vi "Begin.vi"(8 "error in":errorcluster) -> (0 "error out":errorcluster)   [LabVIEW 2018]
doc: "Called before other user functions, this VI is expected to open initial I/O refnums, load in file data, and do all program initialization. Notice that the <B>error out</B> terminal is simply used for data flow. Wiring it to other structures or subVIs ensures that this VI runs first."
uses:
  <vilib>/Rock Robotics/WPI/DriverStation/WPI_DriverStationRobotMode2.ctl
  <vilib>/Rock Robotics/WPI/Joystick/WPI_JoystickDeviceEnum.ctl
  <vilib>/Rock Robotics/WPI/Solenoid/WPI_SolenoidChannel.ctl
  <vilib>/Rock Robotics/WPI/ThirdParty/Phoenix-LabVIEW/Motor Controller/Controls/CTRE_Phoenix_MotorControl_ControlMode.ctl
  <vilib>/Rock Robotics/WPI/SafetyOutput/WPI_SafetyOutputConfigMenu.ctl
  <vilib>/Rock Robotics/SystemInterfaces/DIO/FPGA_DIOChannel.ctl
  Robot Global Data.vi
  <vilib>/Rock Robotics/Network Tables/NT Write String Array.vi
  <vilib>/Rock Robotics/WPI/Solenoid/WPI_SolenoidOpenSingle.vi
  <vilib>/Rock Robotics/WPI/RobotDrive/WPI_RobotDriveOpen2MotorWithExistingMotors.vi
  <vilib>/Rock Robotics/WPI/RobotDrive/WPI_RobotDriveOpen4MotorWithExistingMotors.vi
  <vilib>/Rock Robotics/WPI/Counter/WPI_CounterDigitalInputToDigitalSource.vi
  <vilib>/Rock Robotics/WPI/Utilities/WPI_GetSetVariantRefNum.vi
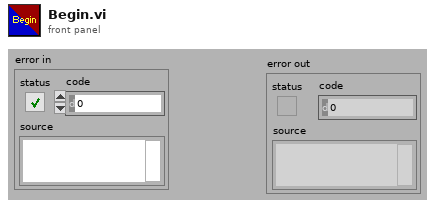
[diagram p1: front panel]
types:
  T1 = typedef "FPGA_DIOChannel.ctl" = enum8{"DIO 0", "DIO 1", "DIO 2", "DIO 3", "DIO 4", "DIO 5", "DIO 6", "DIO 7", "DIO 8", "DIO 9", "DIO MXP 0", "DIO MXP 1", "DIO MXP 2", "DIO MXP 3", "DIO MXP 4", "DIO MXP 5", "DIO MXP 6", "DIO MXP 7", "DIO MXP 8", "DIO MXP 9", "DIO MXP 10", "DIO MXP 11", "DIO MXP 12", "DIO MXP 13", "DIO MXP 14", "DIO MXP 15", "SPI Port CS1", "SPI Port CS2", "SPI Port CS3", "SPI Port MISO", "SPI Port MOSI", "Invalid"}
  T2 = typedef "CTRE_Phoenix_MotorControl_ControlMode.ctl" = u16
  T3 = typedef "WPI_SafetyOutputConfigMenu.ctl" = enum16{"Enable", "Disable"}
  T4 = typedef "WPI_JoystickDeviceEnum.ctl" = enum16{"USB 0", "USB 1", "USB 2", "USB 3", "USB 4", "USB 5"}
  T5 = typedef "WPI_SolenoidChannel.ctl" = enum8{"Solenoid 0", "Solenoid 1", "Solenoid 2", "Solenoid 3", "Solenoid 4", "Solenoid 5", "Solenoid 6", "Solenoid 7", "Invalid"}
  T6 = typedef "WPI_DriverStationRobotMode2.ctl" = enum16{"Autonomous Disabled", "Autonomous Enabled", "Teleop Disabled", "Teleop Enabled", "Disconnected", "Finish", "Test Disabled", "Test Enabled", "Emergency Stopped"}
  T7 = typedef "WPI_MotorControlDeviceRef.ctl" = cluster{"DeviceStatus":errorcluster, "Type":T8, "PWM":cluster{"PWM Channel":T9, "DeadBand":T10}, "CAN":cluster{"Device Number":u8, "SetOutput VI Ref":variant, "GetOutput VI Ref":variant, "Enable VI Ref":variant, "Disable VI Ref":variant, "Data":variant}, "Invert":bool, "DIO PWM":cluster{"PWM \"Enable\" Channel":T9, "DIOChannel":T1, "PWM Rate":dbl}}
  T8 = typedef "WPI_MotorControlType.ctl" = enum16{"PWM", "CAN", "DIO PWM"}
  T9 = typedef "FPGA_DIOPWMChannel.ctl" = enum8{"PWM 0", "PWM 1", "PWM 2", "PWM 3", "PWM 4", "PWM 5", "PWM 6", "PWM 7", "PWM 8", "PWM 9", "PWM MXP 0", "PWM MXP 1", "PWM MXP 2", "PWM MXP 3", "PWM MXP 4", "PWM MXP 5", "PWM MXP 6", "PWM MXP 7", "PWM MXP 8", "PWM MXP 9", "Invalid"}
  T10 = typedef "WPI_PWMDeadband.ctl" = cluster{"Name":string, "maxPositivePwm":i32, "minPositivePwm":i32, "centerPwm":i32, "maxNegativePwm":i32, "minNegativePwm":i32, "angularRange":u16}
  T11 = typedef "WPI_RobotDriveDevRef.ctl" = cluster{"DevStatus":errorcluster, "Motors[]":T7[], "Square Inputs":bool, "Max Output":dbl}
  T12 = typedef "WPI_CompressorDevRef.ctl" = cluster{"DevStatus":errorcluster, "Pneumatics Control Module":u8}
  T13 = typedef "WPI_JoystickDevRef.ctl" = cluster{"Device":T4}
  T14 = typedef "WPI_DigitalInputDevRef.ctl" = cluster{"DevStatus":errorcluster, "DIO Channel":T1}
  T15 = typedef "WPI_SolenoidDevRef.ctl" = cluster{"DevStatus":errorcluster, "Pneumatics Control Module":u8, "Forward Solenoid Channel":T5, "Reverse Solenoid Channel":T5}
  T16 = typedef "FPGA_CounterEncoderSourceConvertionLVSourceType.ctl" = cluster{"DevStatus":errorcluster, "AnalogTriggerMode?":bool, "DigitalMode":cluster{"DIO Channel":T17}, "AnalogTriggerMode":cluster{"AnalogTriggerIndex":T18, "OutputType":T19}}
  T17 = typedef "FPGA_DIODigitalSourceChannel.ctl" = enum8{"DIO 0", "DIO 1", "DIO 2", "DIO 3", "DIO 4", "DIO 5", "DIO 6", "DIO 7", "DIO 8", "DIO 9", "DIO MXP 0", "DIO MXP 1", "DIO MXP 2", "DIO MXP 3", "DIO MXP 4", "DIO MXP 5", "DIO MXP 6", "DIO MXP 7", "DIO MXP 8", "DIO MXP 9", "DIO MXP 10", "DIO MXP 11", "DIO MXP 12", "DIO MXP 13", "DIO MXP 14", "DIO MXP 15", "SPI Port CS1", "SPI Port CS2", "SPI Port CS3", "SPI Port MISO", "SPI Port MOSI", "Disabled"}
  T18 = typedef "FPGA_AnalogTriggerIndex.ctl" = enum8{"Trig 0", "Trig 1", "Trig 2", "Trig 3", "Trig 4", "Trig 5", "Trig 6", "Trig 7", "Invalid"}
  T19 = typedef "FPGA_AnalogTriggerOutType.ctl" = enum16{"InWindow", "TriggerState", "Rising", "Falling"}
  T20 = typedef "WPI_EncoderDevRef.ctl" = cluster{"DevStatus":errorcluster, "EncoderIndex":T21, "CounterIndex":T22, "DistancePerCount":dbl, "Decoding Type":T23}
  T21 = typedef "FPGA_EncoderIdx.ctl" = enum8{"Enc 0", "Enc 1", "Enc 2", "Enc 3", "Enc 4", "Enc 5", "Enc 6", "Enc 7", "Invalid"}
  T22 = typedef "FPGA_CounterCtrSystemIndex.ctl" = enum8{"Ctr 0", "Ctr 1", "Ctr 2", "Ctr 3", "Ctr 4", "Ctr 5", "Ctr 6", "Ctr 7", "Invalid"}
  T23 = typedef "WPI_EncoderType.ctl" = enum16{"1x", "2x", "4x"}
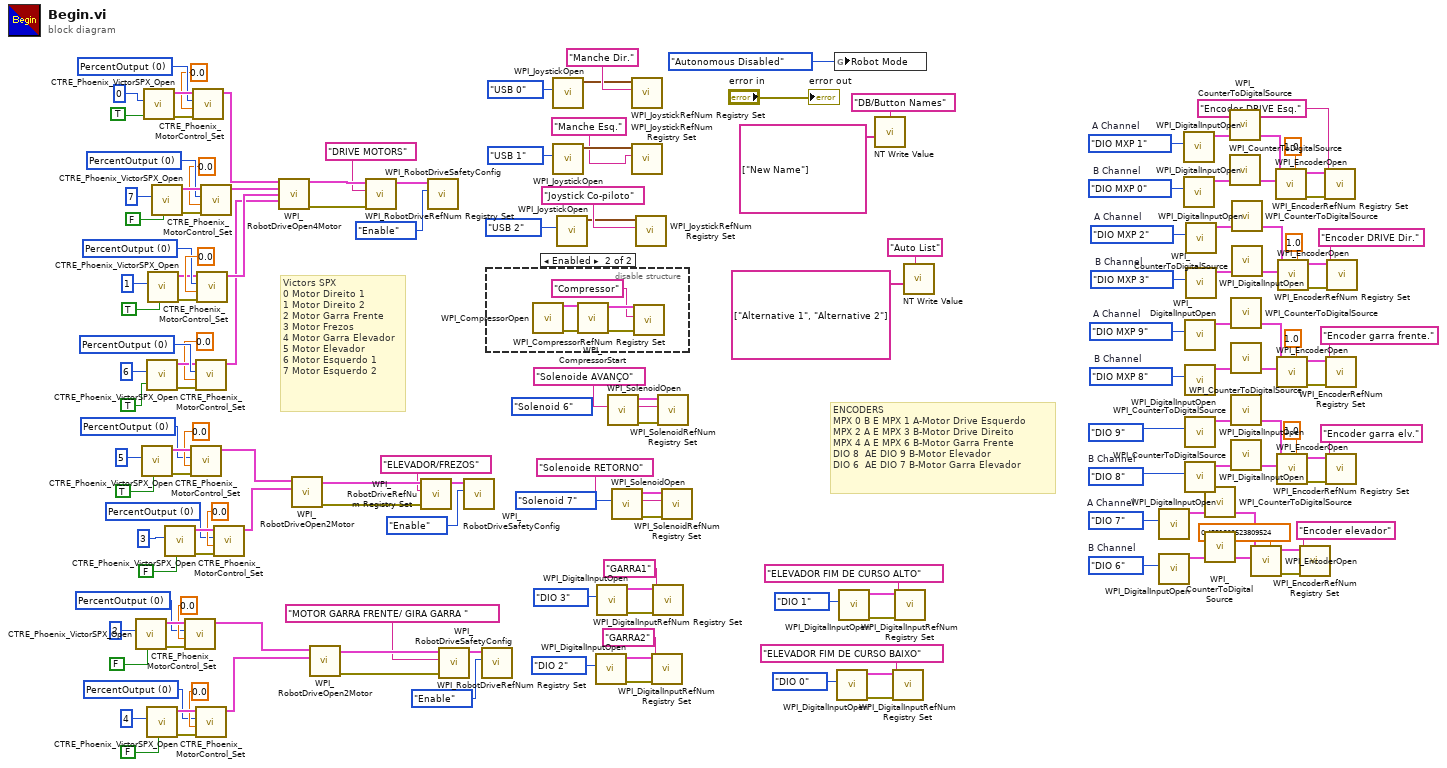
[diagram p0: block diagram]
diagram:
  w15 = FPGA_DIOChannel."DIO MXP 8"  # B Channel
  w14 = FPGA_DIOChannel."DIO MXP 9"  # A Channel
  w16 = FPGA_DIOChannel."DIO 6"  # B Channel
  w17 = FPGA_DIOChannel."DIO 7"  # A Channel
  w35 = FPGA_DIOChannel."DIO MXP 3"  # B Channel
  w34 = FPGA_DIOChannel."DIO MXP 2"  # A Channel
  w45 = FPGA_DIOChannel."DIO MXP 0"  # B Channel
  w44 = FPGA_DIOChannel."DIO MXP 1"  # A Channel
  w54 = FPGA_DIOChannel."DIO 8"  # B Channel
  w82 = T2 0 items=["PercentOutput"=0, "Position"=1, "Velocity"=2, "Current"=3, "Follower"=5, "MotionProfile"=6, "MotionMagic"=7, "MotionProfileArc"=10, "Disabled"=15] ("Control Mode")
  w80 = T2 0 items=["PercentOutput"=0, "Position"=1, "Velocity"=2, "Current"=3, "Follower"=5, "MotionProfile"=6, "MotionMagic"=7, "MotionProfileArc"=10, "Disabled"=15] ("Control Mode")
  w84 = T2 0 items=["PercentOutput"=0, "Position"=1, "Velocity"=2, "Current"=3, "Follower"=5, "MotionProfile"=6, "MotionMagic"=7, "MotionProfileArc"=10, "Disabled"=15] ("Control Mode")
  w97 = T2 0 items=["PercentOutput"=0, "Position"=1, "Velocity"=2, "Current"=3, "Follower"=5, "MotionProfile"=6, "MotionMagic"=7, "MotionProfileArc"=10, "Disabled"=15] ("Control Mode")
  w93 = T2 0 items=["PercentOutput"=0, "Position"=1, "Velocity"=2, "Current"=3, "Follower"=5, "MotionProfile"=6, "MotionMagic"=7, "MotionProfileArc"=10, "Disabled"=15] ("Control Mode")
  w119 = T2 0 items=["PercentOutput"=0, "Position"=1, "Velocity"=2, "Current"=3, "Follower"=5, "MotionProfile"=6, "MotionMagic"=7, "MotionProfileArc"=10, "Disabled"=15] ("Control Mode")
  w116 = T2 0 items=["PercentOutput"=0, "Position"=1, "Velocity"=2, "Current"=3, "Follower"=5, "MotionProfile"=6, "MotionMagic"=7, "MotionProfileArc"=10, "Disabled"=15] ("Control Mode")
  w142 = T2 0 items=["PercentOutput"=0, "Position"=1, "Velocity"=2, "Current"=3, "Follower"=5, "MotionProfile"=6, "MotionMagic"=7, "MotionProfileArc"=10, "Disabled"=15] ("Control Mode")
  # "ENCODERS\nMPX 0 B E MPX 1 A-Motor Drive Esquerdo\nMPX 2 A E MPX 3 B-Motor Drive Direito \nMPX 4 A E MPX 6 B-Motor Garra Frente\nDIO 8  AE DIO 9 B-Motor Elevador\nDIO 6  AE DIO 7 B-Motor Garra Elevador"
  # "Victors SPX\n0 Motor Direito 1\n1 Motor Direito 2 \n2 Motor Garra Frente\n3 Motor Frezos \n4 Motor Garra Elevador\n5 Motor Elevador\n6 Motor Esquerdo 1\n7 Motor Esquerdo 2"
  n1 = call <vilib>:"CTRE_Phoenix_VictorSPX_Open.vi"("Invert"=FALSE, "Device Number"=u8 2) -> ("error out"=w101:errorcluster, "CAN Talon SRX Ref"=w100:T7)  [unwired: 8 in]
  n2 = call <vilib>:"CTRE_Phoenix_VictorSPX_Open.vi"("Invert"=TRUE, "Device Number"=u8 5) -> ("error out"=w123:errorcluster, "CAN Talon SRX Ref"=w122:T7)  [unwired: 8 in]
  n3 = call <vilib>:"CTRE_Phoenix_VictorSPX_Open.vi"("Invert"=TRUE, "Device Number"=u8 0) -> ("error out"=w146:errorcluster, "CAN Talon SRX Ref"=w145:T7)  [unwired: 8 in]
  n4 = call <vilib>:"CTRE_Phoenix_VictorSPX_Open.vi"("Invert"=TRUE, "Device Number"=u8 6) -> ("error out"=w78:errorcluster, "CAN Talon SRX Ref"=w79:T7)  [unwired: 8 in]
  n5 = call <vilib>:"CTRE_Phoenix_VictorSPX_Open.vi"("Invert"=FALSE, "Device Number"=u8 4) -> ("error out"=w103:errorcluster, "CAN Talon SRX Ref"=w104:T7)  [unwired: 8 in]
  n6 = call <vilib>:"CTRE_Phoenix_VictorSPX_Open.vi"("Invert"=TRUE, "Device Number"=u8 1) -> ("error out"=w75:errorcluster, "CAN Talon SRX Ref"=w76:T7)  [unwired: 8 in]
  n7 = call <vilib>:"CTRE_Phoenix_VictorSPX_Open.vi"("Invert"=FALSE, "Device Number"=u8 7) -> ("error out"=w86:errorcluster, "CAN Talon SRX Ref"=w85:T7)  [unwired: 8 in]
  n8 = call <vilib>:"CTRE_Phoenix_VictorSPX_Open.vi"("Invert"=FALSE, "Device Number"=u8 3) -> ("error out"=w125:errorcluster, "CAN Talon SRX Ref"=w126:T7)  [unwired: 8 in]
  n9 = call <vilib>:"CTRE_Phoenix_MotorControl_Set.vi"("error in (no error)"=w101, "Output"=0.0, "Control Mode"=w93, "PhoenixMotorControlDevRef"=w100) -> ("PhoenixMotorControlDevRef"=w102:T7)  [unwired: 6 in, 1 out]
  n10 = call <vilib>:"CTRE_Phoenix_MotorControl_Set.vi"("error in (no error)"=w123, "Output"=0.0, "Control Mode"=w116, "PhoenixMotorControlDevRef"=w122) -> ("PhoenixMotorControlDevRef"=w124:T7)  [unwired: 6 in, 1 out]
  n11 = call <vilib>:"CTRE_Phoenix_MotorControl_Set.vi"("error in (no error)"=w146, "Output"=0.0, "Control Mode"=w142, "PhoenixMotorControlDevRef"=w145) -> ("PhoenixMotorControlDevRef"=w144:T7)  [unwired: 6 in, 1 out]
  n12 = call <vilib>:"CTRE_Phoenix_MotorControl_Set.vi"("error in (no error)"=w78, "Output"=0.0, "Control Mode"=w82, "PhoenixMotorControlDevRef"=w79) -> ("PhoenixMotorControlDevRef"=w139:T7)  [unwired: 6 in, 1 out]
  n13 = call <vilib>:"CTRE_Phoenix_MotorControl_Set.vi"("error in (no error)"=w103, "Output"=0.0, "Control Mode"=w97, "PhoenixMotorControlDevRef"=w104) -> ("PhoenixMotorControlDevRef"=w105:T7)  [unwired: 6 in, 1 out]
  n14 = call <vilib>:"CTRE_Phoenix_MotorControl_Set.vi"("error in (no error)"=w75, "Output"=0.0, "Control Mode"=w80, "PhoenixMotorControlDevRef"=w76) -> ("PhoenixMotorControlDevRef"=w140:T7)  [unwired: 6 in, 1 out]
  n15 = call <vilib>:"CTRE_Phoenix_MotorControl_Set.vi"("error in (no error)"=w86, "Output"=0.0, "Control Mode"=w84, "PhoenixMotorControlDevRef"=w85) -> ("PhoenixMotorControlDevRef"=w143:T7)  [unwired: 6 in, 1 out]
  n16 = call <vilib>:"CTRE_Phoenix_MotorControl_Set.vi"("error in (no error)"=w125, "Output"=0.0, "Control Mode"=w119, "PhoenixMotorControlDevRef"=w126) -> ("PhoenixMotorControlDevRef"=w127:T7)  [unwired: 6 in, 1 out]
  n17 = call-poly <vilib>:"WPI_RobotDriveOpen4Motor.vi"("Rear Left Motor Dev Ref"=w144, "Rear Right Motor Dev Ref"=w143, "Front Left Motor Dev Ref"=w140, "Front Right Motor Dev Ref"=w139) -> ("RobotDriveDevRef"=w160:T11, "error out"=w158:errorcluster)  [unwired: 10 in]
  n18 = call-poly <vilib>:"WPI_RobotDriveOpen2Motor.vi"("Right Motor Dev Ref"=w127, "Left Motor Dev Ref"=w124) -> ("error out"=w130:errorcluster, "RobotDriveDevRef"=w129:T11)  [unwired: 8 in]
  n19 = call-poly <vilib>:"WPI_RobotDriveOpen2Motor.vi"("Right Motor Dev Ref"=w105, "Left Motor Dev Ref"=w102) -> ("error out"=w108:errorcluster, "RobotDriveDevRef"=w107:T11)  [unwired: 8 in]
  n20 = call <vilib>:"WPI_RobotDriveRefNum Registry Set.vi"("error in (no error)"=w158, "refnum name"="DRIVE MOTORS", "RobotDriveDevRef"=w160) -> ("RobotDriveDevRef"=w157:T11)  [unwired: 1 in, 7 out]
  n21 = call <vilib>:"WPI_RobotDriveRefNum Registry Set.vi"("error in (no error)"=w130, "refnum name"="ELEVADOR/FREZOS", "RobotDriveDevRef"=w129) -> ("RobotDriveDevRef"=w128:T11)  [unwired: 1 in, 7 out]
  n22 = call <vilib>:"WPI_RobotDriveSafetyConfig.vi"("mode"=WPI_SafetyOutputConfigMenu."Enable", "RobotDriveDevRef"=w157) -> ()  [unwired: 8 in, 2 out]
  n23 = call <vilib>:"WPI_RobotDriveRefNum Registry Set.vi"("error in (no error)"=w108, "refnum name"="MOTOR GARRA FRENTE/ GIRA GARRA ", "RobotDriveDevRef"=w107) -> ("RobotDriveDevRef"=w106:T11)  [unwired: 1 in, 7 out]
  n24 = call <vilib>:"WPI_RobotDriveSafetyConfig.vi"("mode"=WPI_SafetyOutputConfigMenu."Enable", "RobotDriveDevRef"=w128) -> ()  [unwired: 8 in, 2 out]
  n25 = call <vilib>:"WPI_RobotDriveSafetyConfig.vi"("mode"=WPI_SafetyOutputConfigMenu."Enable", "RobotDriveDevRef"=w106) -> ()  [unwired: 8 in, 2 out]
  n26 = disable-structure shown="Enabled" {
    frame Disabled {
    }
    frame Enabled {
      n27 = call <vilib>:"WPI_CompressorOpen.vi"() -> ("CompressorDevRef"=w163:T12, "error out"=w162:errorcluster)  [unwired: 14 in]
      n28 = call <vilib>:"WPI_CompressorStart.vi"("error in (no error)"=w162, "CompressorDevRef"=w163) -> ("error out"=w165:errorcluster, "CompressorDevRef"=w164:T12)  [unwired: 8 in]
      n29 = call <vilib>:"WPI_CompressorRefNum Registry Set.vi"("error in (no error)"=w165, "refnum name"="Compressor", "CompressorDevRef"=w164) -> ()  [unwired: 7 in, 2 out]
    }
  }
  n30 = call <vilib>:"WPI_JoystickOpen.vi"("JoystickDevice"=WPI_JoystickDeviceEnum."USB 0") -> ("JoystickDevRef"=w153:T13)  [unwired: 10 in]
  n31 = call <vilib>:"WPI_JoystickOpen.vi"("JoystickDevice"=WPI_JoystickDeviceEnum."USB 1") -> ("JoystickDevRef"=w113:T13)  [unwired: 10 in]
  n32 = call <vilib>:"WPI_JoystickOpen.vi"("JoystickDevice"=WPI_JoystickDeviceEnum."USB 2") -> ("JoystickDevRef"=w110:T13)  [unwired: 10 in]
  n33 = call <vilib>:"WPI_DigitalInputOpen.vi"("DIO Channel"=FPGA_DIOChannel."DIO 2") -> ("error out"=w66:errorcluster, "DigitalInputDevRef"=w65:T14)  [unwired: 1 in, 8 out]
  n34 = call <vilib>:"WPI_DigitalInputOpen.vi"("DIO Channel"=FPGA_DIOChannel."DIO 3") -> ("error out"=w70:errorcluster, "DigitalInputDevRef"=w69:T14)  [unwired: 1 in, 8 out]
  n35 = call-poly <vilib>:"WPI_SolenoidOpen.vi"("Solenoid Channel"=WPI_SolenoidChannel."Solenoid 6" ("Forward Solenoid Channel")) -> ("error out"=w138:errorcluster, "SolenoidDevRef"=w137:T15)  [unwired: 9 in]
  n36 = call-poly <vilib>:"WPI_SolenoidOpen.vi"("Solenoid Channel"=WPI_SolenoidChannel."Solenoid 7" ("Forward Solenoid Channel")) -> ("error out"=w131:errorcluster, "SolenoidDevRef"=w132:T15)  [unwired: 9 in]
  n37 = call <vilib>:"WPI_JoystickRefNum Registry Set.vi"("refnum name"="Manche Dir.", "JoystickDevRef"=w153) -> ()  [unwired: 8 in, 2 out]
  n38 = call <vilib>:"WPI_JoystickRefNum Registry Set.vi"("refnum name"="Manche Esq.", "JoystickDevRef"=w113) -> ()  [unwired: 8 in, 2 out]
  n39 = call <vilib>:"WPI_JoystickRefNum Registry Set.vi"("refnum name"="Joystick Co-piloto", "JoystickDevRef"=w110) -> ()  [unwired: 8 in, 2 out]
  n40 = call <vilib>:"WPI_DigitalInputRefNum Registry Set.vi"("error in (no error)"=w66, "refnum name"="GARRA2", "DigitalInputDevRef"=w65) -> ()  [unwired: 7 in, 2 out]
  n41 = call <vilib>:"WPI_DigitalInputRefNum Registry Set.vi"("error in (no error)"=w70, "refnum name"="GARRA1", "DigitalInputDevRef"=w69) -> ()  [unwired: 7 in, 2 out]
  n42 = call <vilib>:"WPI_SolenoidRefNum Registry Set.vi"("error in (no error)"=w138, "refnum name"="Solenoide AVANÇO", "SolenoidDevRef"=w137) -> ()  [unwired: 7 in, 2 out]
  n43 = call <vilib>:"WPI_SolenoidRefNum Registry Set.vi"("error in (no error)"=w131, "refnum name"="Solenoide RETORNO", "SolenoidDevRef"=w132) -> ()  [unwired: 7 in, 2 out]
  n44 = global write "Robot Global Data.vi" "Robot Mode"(WPI_DriverStationRobotMode2."Autonomous Disabled" ("Robot Mode")) -> ()
  n45 = call <vilib>:"WPI_DigitalInputOpen.vi"("DIO Channel"=FPGA_DIOChannel."DIO 0") -> ("error out"=w58:errorcluster, "DigitalInputDevRef"=w57:T14)  [unwired: 1 in, 8 out]
  n46 = call <vilib>:"WPI_DigitalInputOpen.vi"("DIO Channel"=FPGA_DIOChannel."DIO 1") -> ("error out"=w62:errorcluster, "DigitalInputDevRef"=w61:T14)  [unwired: 1 in, 8 out]
  n47 = call-poly <vilib>:"NT Write Value.vi"("String Array"=string[] ["New Name"], "Name"="DB/Button Names") -> ()  [unwired: 9 in, 1 out]
  n48 = call <vilib>:"WPI_DigitalInputRefNum Registry Set.vi"("error in (no error)"=w58, "refnum name"="ELEVADOR FIM DE CURSO BAIXO", "DigitalInputDevRef"=w57) -> ()  [unwired: 7 in, 2 out]
  n49 = call <vilib>:"WPI_DigitalInputRefNum Registry Set.vi"("error in (no error)"=w62, "refnum name"="ELEVADOR FIM DE CURSO ALTO", "DigitalInputDevRef"=w61) -> ()  [unwired: 7 in, 2 out]
  n50 = call-poly <vilib>:"NT Write Value.vi"("String Array"=string[] ["Alternative 1", "Alternative 2"], "Name"="Auto List") -> ()  [unwired: 9 in, 1 out]
  n51 = call <vilib>:"WPI_DigitalInputOpen.vi"("DIO Channel"=w17) -> ("DigitalInputDevRef"=w20:T14)  [unwired: 1 in, 9 out]
  n52 = call <vilib>:"WPI_DigitalInputOpen.vi"("DIO Channel"=w16) -> ("DigitalInputDevRef"=w19:T14)  [unwired: 1 in, 9 out]
  n53 = call <vilib>:"WPI_DigitalInputOpen.vi"("DIO Channel"=w44) -> ("DigitalInputDevRef"=w41:T14)  [unwired: 1 in, 9 out]
  n54 = call <vilib>:"WPI_DigitalInputOpen.vi"("DIO Channel"=w45) -> ("DigitalInputDevRef"=w42:T14)  [unwired: 1 in, 9 out]
  n55 = call <vilib>:"WPI_DigitalInputOpen.vi"("DIO Channel"=w14) -> ("DigitalInputDevRef"=w11:T14)  [unwired: 1 in, 9 out]
  n56 = call <vilib>:"WPI_DigitalInputOpen.vi"("DIO Channel"=w15) -> ("DigitalInputDevRef"=w12:T14)  [unwired: 1 in, 9 out]
  n57 = call <vilib>:"WPI_DigitalInputOpen.vi"("DIO Channel"=FPGA_DIOChannel."DIO 9") -> ("DigitalInputDevRef"=w51:T14)  [unwired: 1 in, 9 out]
  n58 = call <vilib>:"WPI_DigitalInputOpen.vi"("DIO Channel"=w54) -> ("DigitalInputDevRef"=w52:T14)  [unwired: 1 in, 9 out]
  n59 = call <vilib>:"WPI_DigitalInputOpen.vi"("DIO Channel"=w34) -> ("DigitalInputDevRef"=w31:T14)  [unwired: 1 in, 9 out]
  n60 = call <vilib>:"WPI_DigitalInputOpen.vi"("DIO Channel"=w35) -> ("DigitalInputDevRef"=w32:T14)  [unwired: 1 in, 9 out]
  n61 = call-poly <vilib>:"WPI_CounterToDigitalSource.vi"("DigitalInputDevRef"=w20) -> ("Digital Source"=w21:T16)  [unwired: 6 out]
  n62 = call-poly <vilib>:"WPI_CounterToDigitalSource.vi"("DigitalInputDevRef"=w19) -> ("Digital Source"=w18:T16)  [unwired: 6 out]
  n63 = call-poly <vilib>:"WPI_CounterToDigitalSource.vi"("DigitalInputDevRef"=w41) -> ("Digital Source"=w40:T16)  [unwired: 6 out]
  n64 = call-poly <vilib>:"WPI_CounterToDigitalSource.vi"("DigitalInputDevRef"=w42) -> ("Digital Source"=w43:T16)  [unwired: 6 out]
  n65 = call-poly <vilib>:"WPI_CounterToDigitalSource.vi"("DigitalInputDevRef"=w11) -> ("Digital Source"=w10:T16)  [unwired: 6 out]
  n66 = call-poly <vilib>:"WPI_CounterToDigitalSource.vi"("DigitalInputDevRef"=w12) -> ("Digital Source"=w13:T16)  [unwired: 6 out]
  n67 = call-poly <vilib>:"WPI_CounterToDigitalSource.vi"("DigitalInputDevRef"=w51) -> ("Digital Source"=w50:T16)  [unwired: 6 out]
  n68 = call-poly <vilib>:"WPI_CounterToDigitalSource.vi"("DigitalInputDevRef"=w52) -> ("Digital Source"=w53:T16)  [unwired: 6 out]
  n69 = call-poly <vilib>:"WPI_CounterToDigitalSource.vi"("DigitalInputDevRef"=w31) -> ("Digital Source"=w30:T16)  [unwired: 6 out]
  n70 = call-poly <vilib>:"WPI_CounterToDigitalSource.vi"("DigitalInputDevRef"=w32) -> ("Digital Source"=w33:T16)  [unwired: 6 out]
  n71 = call <vilib>:"WPI_EncoderOpen.vi"("DistancePerCount"=0.4331809523809524, "BSource"=w18, "ASource"=w21) -> ("error out"=w22:errorcluster, "EncoderDevRef"=w23:T20)  [unwired: 5 in, 2 out]
  n72 = call <vilib>:"WPI_EncoderOpen.vi"("DistancePerCount"=1.0, "BSource"=w43, "ASource"=w40) -> ("error out"=w39:errorcluster, "EncoderDevRef"=w38:T20)  [unwired: 5 in, 2 out]
  n73 = call <vilib>:"WPI_EncoderOpen.vi"("DistancePerCount"=1.0, "BSource"=w13, "ASource"=w10) -> ("error out"=w9:errorcluster, "EncoderDevRef"=w8:T20)  [unwired: 5 in, 2 out]
  n74 = call <vilib>:"WPI_EncoderOpen.vi"("DistancePerCount"=1.0, "BSource"=w53, "ASource"=w50) -> ("error out"=w49:errorcluster, "EncoderDevRef"=w48:T20)  [unwired: 5 in, 2 out]
  n75 = call <vilib>:"WPI_EncoderOpen.vi"("DistancePerCount"=1.0, "BSource"=w33, "ASource"=w30) -> ("error out"=w29:errorcluster, "EncoderDevRef"=w28:T20)  [unwired: 5 in, 2 out]
  n76 = call <vilib>:"WPI_EncoderRefNum Registry Set.vi"("error in (no error)"=w22, "refnum name"="Encoder elevador", "EncoderDevRef"=w23) -> ()  [unwired: 7 in, 2 out]
  n77 = call <vilib>:"WPI_EncoderRefNum Registry Set.vi"("error in (no error)"=w39, "refnum name"="Encoder DRIVE Esq.", "EncoderDevRef"=w38) -> ()  [unwired: 7 in, 2 out]
  n78 = call <vilib>:"WPI_EncoderRefNum Registry Set.vi"("error in (no error)"=w9, "refnum name"="Encoder garra frente.", "EncoderDevRef"=w8) -> ()  [unwired: 7 in, 2 out]
  n79 = call <vilib>:"WPI_EncoderRefNum Registry Set.vi"("error in (no error)"=w49, "refnum name"="Encoder garra elv.", "EncoderDevRef"=w48) -> ()  [unwired: 7 in, 2 out]
  n80 = call <vilib>:"WPI_EncoderRefNum Registry Set.vi"("error in (no error)"=w29, "refnum name"="Encoder DRIVE Dir.", "EncoderDevRef"=w28) -> ()  [unwired: 7 in, 2 out]
  "error out" <- "error in"
